vi "format_json_string.vi"(8 "error in (no error)":errorcluster, 11 "log_entry":T1 {"datetime" format="%<%x %.3X>T"}) -> (0 "error out":errorcluster, 2 "json":string)   [LabVIEW 2021, in "json.provider.lvclass"]
uses:
  json.provider.lvclass
  system.logging/log_entry.ctl
  system.logging/severity.ctl
  json_compatibility.ctl
  json.provider.lvclass/json.provider.ctl
  system.logging/system.logging.lvclass
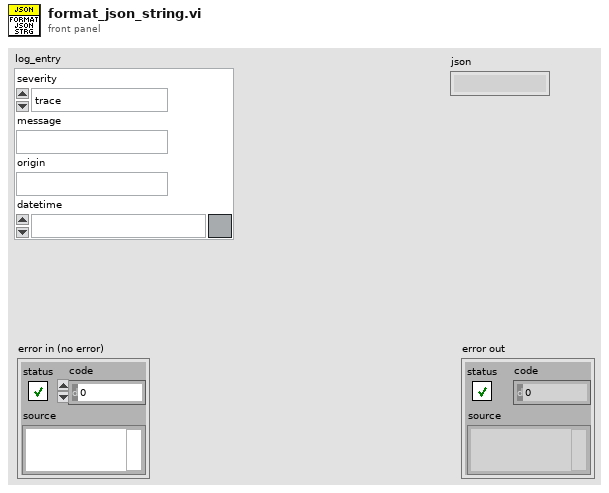
[diagram p1: front panel]
types:
  T1 = typedef "system.logging.lvclass/log_entry.ctl" = cluster{"severity":T2, "message":string, "origin":string, "datetime":timestamp}
  T2 = typedef "system.logging.lvclass/severity.ctl" = enum8{"trace", "debug", "info", "warning", "error"}
  T3 = typedef "json.provider.lvclass/json_compatibility.ctl" = cluster{"datetime":string, "severity":string, "origin":string, "message":string}
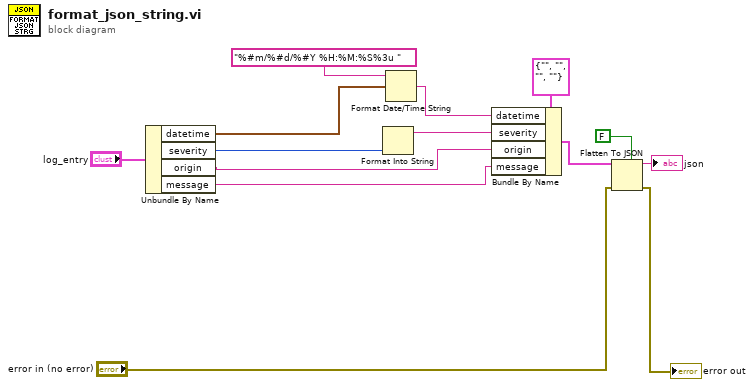
[diagram p0: block diagram]
diagram:
  n1 = Unbundle By Name("log_entry") -> ("datetime"=w12:timestamp, "severity"=w11:T2, "origin"=w7:string, "message"=w6:string)
  n2 = Format Into String(w11) -> (resulting string=w8:string)  [unwired: 3 in, 1 out]
  n3 = Format Date/Time String(time format string (%c)="%#m/%#d/%#Y %H:%M:%S%3u ", seconds (now)=w12) -> (date/time string=w9:string)  [unwired: 1 in]
  n4 = Bundle By Name(cluster=T3 {"datetime"="", "severity"="", "origin"="", "message"=""} ("json_compatibility"), "datetime"=w9, "severity"=w8, "origin"=w7, "message"=w6) -> (w3:T3)
  n5 = Flatten To JSON(enable LabVIEW extensions? (T)=FALSE, anything=w3, error in (no error)="error in (no error)") -> (JSON string=→"json":string, 11:→"error out":errorcluster)
